vi "Right.vi"(1 "背景":dbl[][](array[numeric]), 2 "方块":dbl[][](array[numeric]), 3 "point":cluster{"x":i16, "y":i16} caption="位置") -> (0 "point 2":cluster{"x":i16, "y":i16} caption="新位置")   [LabVIEW 2016]
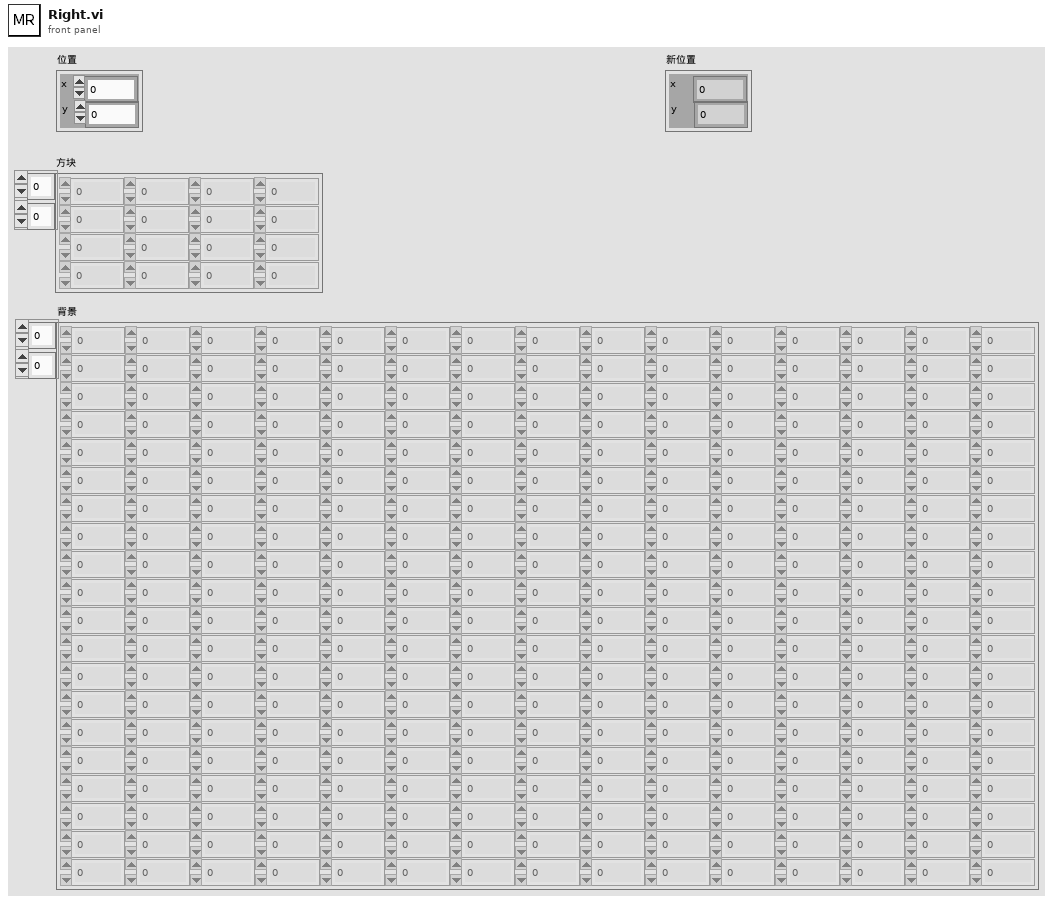
[diagram p1: front panel]
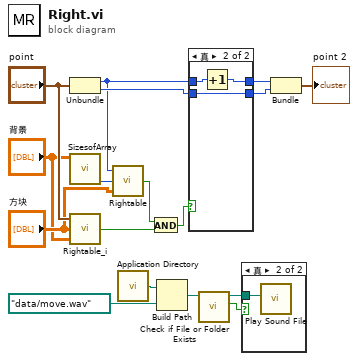
[diagram p0: block diagram]
diagram:
  n1 = Unbundle("point") -> ("x"=w12:i16, "y"=w16:i16)
  n2 = call "SizesofArray.vi"("数组"="背景") -> ("NumCols_r"=w1:i32)  [unwired: 7 in, 3 out]
  n3 = call "Rightable_i.vi"("背景"="背景", "方块"="方块", "point"="point") -> ("输出"=w8:bool)
  n4 = call "Rightable.vi"("方块"="方块", "宽度"=w1, "x"=w12) -> ("输出"=w11:bool)
  n5 = call <vilib>:"Application Directory.vi"() -> ("Application Directory"=w6:path)
  n6 = And(x=w11, y=w8) -> (x .and. y?=w17:bool)
  n7 = Build Path(base path=w6, name or relative path=path "data/move.wav") -> (appended path=w5:path)
  n8 = case shown="真" w17 {
    tunnel: w16 -> [w18 w22]
    tunnel: w12 -> [w19 w21]
    tunnel: [w19 w20] -> w15
    tunnel: [w18 w22] -> w14
    frame False {
    }
    frame True {
      n9 = Increment(x=w21) -> (x+1=w20:i16)
    }
  }
  n10 = call <vilib>:"Check if File or Folder Exists.vi"("path"=w5) -> ("file or folder exists?"=w4:bool, "dup path"=w3:path)  [unwired: 8 in, 1 out]
  n11 = case shown="真" w4 {
    tunnel: w3 -> [_ w23]
    frame False {
    }
    frame True {
      n12 = call <vilib>:"Play Sound File.vi"("path"=w23) -> ()  [unwired: 9 in, 2 out]
    }
  }
  n13 = Bundle("x"=w15, "y"=w14) -> (→"point 2":cluster{"x":i16, "y":i16})  [unwired: 1 in]
